vi "hmi_initialize.vi"(5 "hmi_references":T1, 7 "post_installer []":refnum<class "lv-post-installer.lvclass">[](array[class]), 8 "error in (no error)":errorcluster) -> (0 "error out":errorcluster)   [LabVIEW 2015, in "lv-post-installer-interface.lvlib"]
uses:
  lv-post-installer-interface.lvlib
  _controls/hmi_references.ctl
  lv-post-installer/public/classes/lv-post-installer/lv-post-installer.lvclass
  _controls/tab_control.ctl
  _controls/navigation.ctl
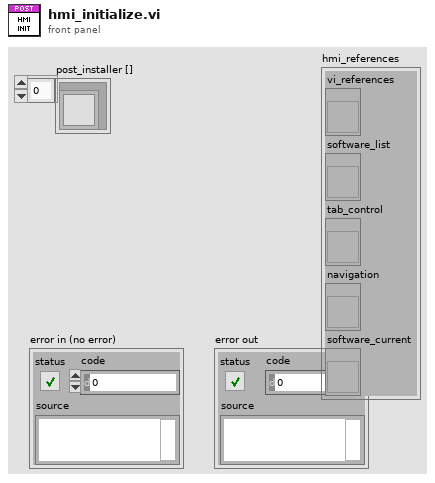
[diagram p1: front panel]
types:
  T1 = typedef "lv-post-installer-interface.lvlib/hmi_references.ctl" = cluster{"vi_references":refnum<vi>, "software_list":refnum<vi>, "tab_control":refnum<vi>, "navigation":refnum<vi>, "software_current":refnum<vi>}
  T2 = typedef "lv-post-installer-interface.lvlib/navigation.ctl" = enum32{"auxiliary", "automatic", "manual"}
  T3 = typedef "lv-post-installer-interface.lvlib/tab_control.ctl" = enum32{"automatic", "manual", "auxiliary"}
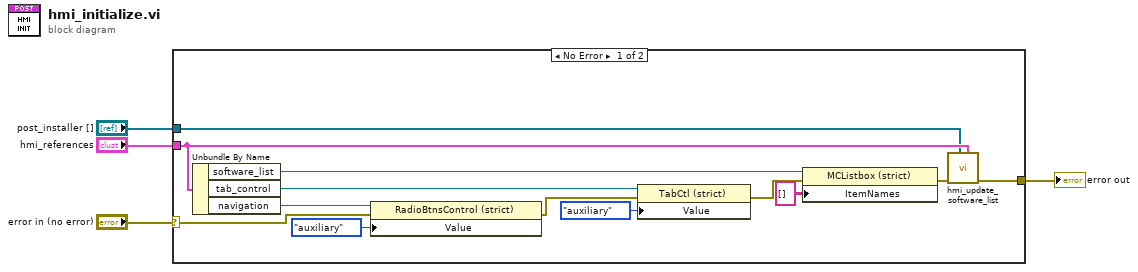
[diagram p0: block diagram]
diagram:
  n1 = case shown="No Error" "error in (no error)" {
    selector: "error in (no error)" -> [w14 w18]
    tunnel: [w7 w18] -> w3
    tunnel: "hmi_references" -> [w6 _]
    tunnel: "post_installer []" -> [w5 _]
    frame No Error {
      n2 = Unbundle By Name(w6) -> ("software_list"=w11:refnum<vi>, "tab_control"=w10:refnum<vi>, "navigation"=w9:refnum<vi>)
      n3 = property on="Property Node" class="RadioBtnsControl (strict)"(reference=w9, error in=w14, "Value"=navigation."auxiliary" ("navigation")) -> (error out=w15:errorcluster)  [unwired: 1 out]
      n4 = property on="Property Node" class="TabCtl (strict)"(reference=w10, error in=w15, "Value"=tab_control."auxiliary" ("tab_control")) -> (error out=w13:errorcluster)  [unwired: 1 out]
      n5 = property on="Property Node" class="MCListbox (strict)"(reference=w11, error in=w13, "ItemNames"=string[][] [] ("Item Names")) -> (error out=w8:errorcluster)  [unwired: 1 out]
      n6 = call "hmi_update_software_list.vi"("hmi_references"=w6, "post_installer []"=w5, "error in (no error)"=w8) -> ("error out"=w7:errorcluster)  [unwired: 8 in]
    }
    frame Error {
    }
  }
  "error out" <- w3
